vi "Verify Folder Exists and Writable.vi"(8 "error in (no error)":errorcluster, 11 "path in":path) -> (0 "error out":errorcluster, 3 "path out":path)   [LabVIEW 2024, in "DSA_CFG_ACQ.lvlib"]
uses:
  DSA_CFG_ACQ.lvlib
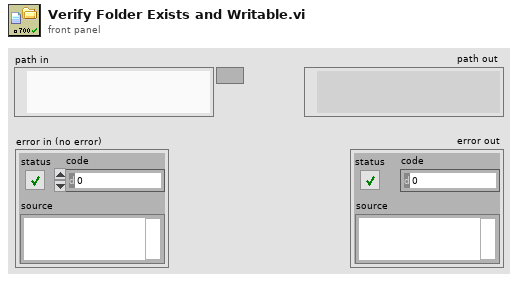
[diagram p1: front panel]
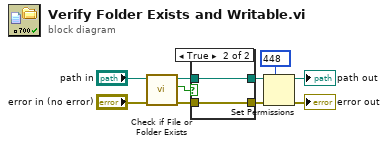
[diagram p0: block diagram]
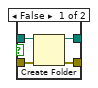
[diagram p2: hidden frame]
diagram:
  n1 = call <vilib>:"Check if File or Folder Exists.vi"("error in (no error)"="error in (no error)", "path"="path in") -> ("error out"=w5:errorcluster, "file or folder exists?"=w1:bool, "dup path"=w3:path)  [unwired: 7 in]
  n2 = case shown="True" w1 {
    tunnel: [w13 w16] -> w2
    tunnel: w3 -> [w14 w16]
    tunnel: w5 -> [w12 w15]
    tunnel: [w11 w15] -> w6
    frame False {
      n3 = Create Folder(path (use dialog)=w14, error in=w12) -> (created path=w13:path, error out=w11:errorcluster)  [unwired: 1 in, 1 out]
    }
    frame True {
    }
  }
  n4 = Set Permissions(7:i16 448 ("permissions"), 8:w6, 11:w2) -> (0:→"error out":errorcluster, 3:→"path out":path)  [unwired: 2 in]
